vi "Magic.vi"(8 "error in":errorcluster, 9 "Path":path, 10 "Visualize VI Ref":refnum<vi>, 11 "Parent VI":refnum<vi>) -> (0 "error out":errorcluster)   [LabVIEW 2016]
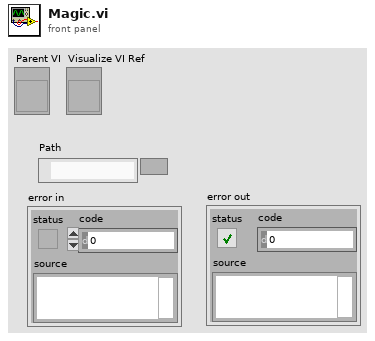
[diagram p1: front panel]
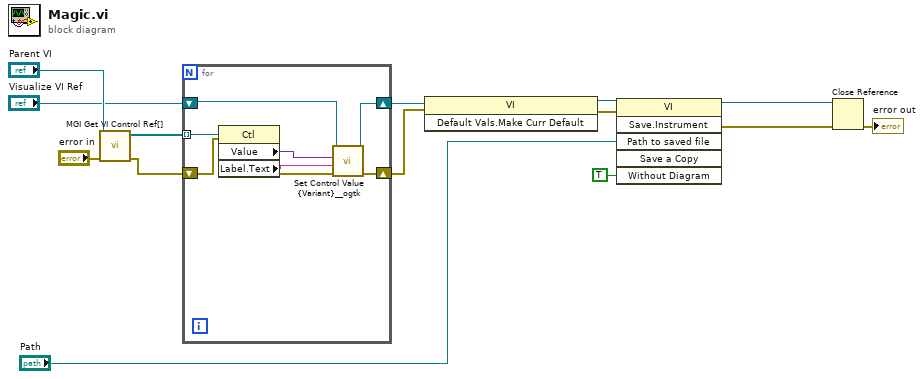
[diagram p0: block diagram]
diagram:
  n1 = call <userlib>:"MGI Get VI Control Ref[].vi"("error in"="error in", "VI (Caller)"="Parent VI") -> ("error out"=w4:errorcluster, "Control[i]"=w13:refnum<vi>[])  [unwired: 6 in, 2 out]
  n2 = for {
    tunnel: w13 -> [w22] mode=indexing
    shift-right: [w18] -> w11
    shift-left: "Visualize VI Ref" -> [w19]
    shift-right: [w15] -> w3
    shift-left: w4 -> [w17]
    n3 = property class="Ctl"(reference=w22, error in=w17) -> (error out=w16:errorcluster, "Value"=w21:variant, "Label.Text"=w20:string)  [unwired: 1 out]
    n4 = call <userlib>:"Set Control Value {Variant}__ogtk.vi"("error in (no error)"=w16, "Control Name (\"\": use variant name)"=w20, "Value"=w21, "VI Refnum"=w19) -> ("error out"=w15:errorcluster, "VI Refnum dup"=w18:refnum<vi>)  [unwired: 6 in]
  }
  n5 = invoke class="VI" method="Default Vals.Make Curr Default"(reference=w11, error in=w3) -> (reference out=w10:refnum<vi>, error out=w6:errorcluster)  [unwired: 1 in, 1 out]
  n6 = invoke class="VI" method="Save.Instrument"(reference=w10, error in=w6, "Path to saved file"="Path", "Without Diagram"=TRUE) -> (reference out=w7:refnum<vi>, error out=w5:errorcluster)  [unwired: 2 in, 4 out]
  n7 = Close Reference(reference=w7, error in (no error)=w5) -> (error out=→"error out":errorcluster)
